vi "SettingsDialog.vi"() -> ()   [LabVIEW 2020]
uses:
  controls/PlayerMode.ctl
panel:
  out "Comment":string
  in  "Cancel Button":bool
  in  "OK Button":bool
  in  "Player 2":T1
  in  "Player 1":T1
  # "Settings"
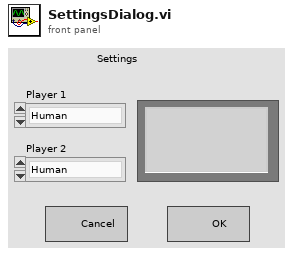
[diagram p1: front panel]
types:
  T1 = typedef "PlayerMode.ctl" = enum16{"Human", "Bot Random", "Bot Intermidiate", "Bot Perfect Play"}
  T2 = typedef "PlayerSettings.ctl" = cluster{"Player 1":T1, "Player 2":T1}
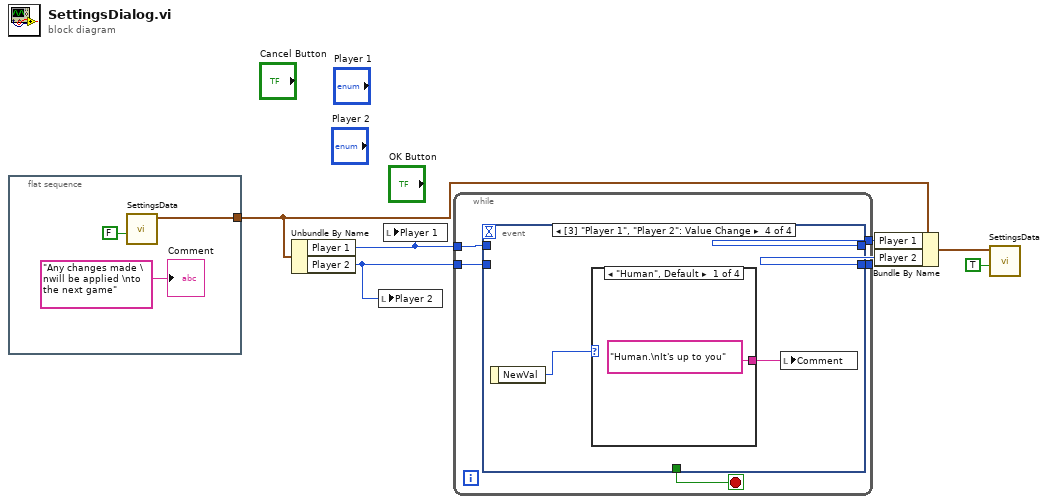
[diagram p0: block diagram]
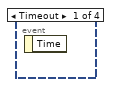
[diagram p2: hidden frame]
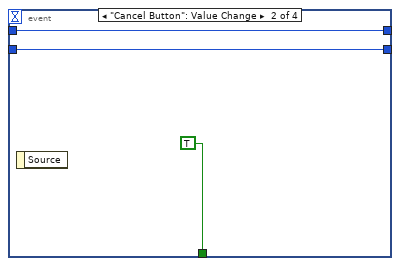
[diagram p3: hidden frame]
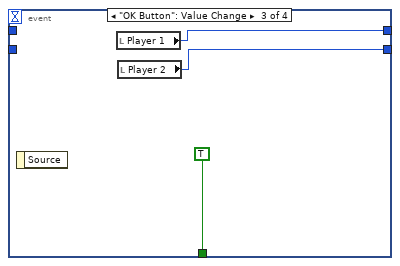
[diagram p4: hidden frame]
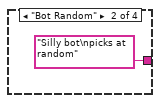
[diagram p5: hidden frame]
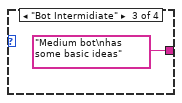
[diagram p6: hidden frame]
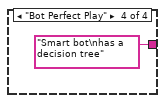
[diagram p7: hidden frame]
diagram:
  n1 = flat-sequence {
    tunnel: [w9] -> w1
    frame #0 {
      n2 = call "SettingsData.vi"("Write (T)/Read (F)"=FALSE) -> ("Settings out"=w9:T2)  [unwired: 10 in]
      "Comment" <- "Any changes made \nwill be applied \nto the next game" ("Comment")
    }
  }
  n3 = Unbundle By Name(w1) -> ("Player 1"=w5:T1, "Player 2"=w4:T1)
  n4 = local write "Player 2"(w4) -> ()
  n5 = local write "Player 1"(w5) -> ()
  n6 = while {
    tunnel: w5 -> [w15]
    tunnel: w4 -> [w14]
    tunnel: [w13] -> w3
    tunnel: [w12] -> w2
    stop <- w11 stop-if-true
    n7 = event shown="[3] \"Player 1\", \"Player 2\": Value Change" {
      selector: _ -> [_ _ _ _]
      dyn-events: _ -> [_ _ _ _]
      timeout: _ -> [_ _ _ _]
      tunnel: w15 -> [_ w18 _ _]
      tunnel: w14 -> [_ w17 _ _]
      tunnel: [_ w18 w21 _] -> w13
      tunnel: [_ w17 w20 _] -> w12
      tunnel: [_ TRUE TRUE _] -> w11
      event Timeout {
        n8 = event-data() -> ()  [unwired: 1 in, 1 out]
      }
      event "Cancel Button": Value Change {
        n9 = event-data() -> ()  [unwired: 1 in, 1 out]
      }
      event "OK Button": Value Change {
        n10 = event-data() -> ()  [unwired: 1 in, 1 out]
        n11 = local read "Player 1"() -> (w21:T1)
        n12 = local read "Player 2"() -> (w20:T1)
      }
      event Value Change {
        n13 = event-data() -> ("NewVal"=w23:T1)  [unwired: 1 in]
        n14 = case shown="\"Human\", Default" w23 {
          tunnel: ["Human.\nIt's up to you" "Silly bot\npicks at random" "Medium bot\nhas some basic ideas" "Smart bot\nhas a decision tree"] -> w22
          frame "Human", Default {
          }
          frame "Bot Random" {
          }
          frame "Bot Intermidiate" {
          }
          frame "Bot Perfect Play" {
          }
        }
        n15 = local write "Comment"(w22) -> ()
      }
    }
  }
  n16 = Bundle By Name(cluster=w1, "Player 1"=w3, "Player 2"=w2) -> (w6:T2)
  n17 = call "SettingsData.vi"("Write (T)/Read (F)"=TRUE, "Settings in"=w6) -> ()  [unwired: 9 in, 1 out]
